vi "Read Math Voltage.vi"(8 "error in (no error)":errorcluster, 11 "VISA resource name":refnum<visa-resource-name>) -> (0 "error out":errorcluster, 2 "amplitude":dbl format="%.2p", 3 "VISA resource name out":refnum<visa-resource-name>)   [LabVIEW 2017]
doc: "You need to run the Initilize.Vi and the Close.vi for the Oscilloscope before and after this Vi. This doens't include those for the sake of runtime."
uses:
  <instrlib>/Tektronix TDS 200 1000 2000 Series/Public/Data/Read (Single Waveform).vi
  <vilib>/measure/mascope.llb/Amplitude and Levels 1 chan.vi
  <instrlib>/Tektronix TDS 200 1000 2000 Series/Tektronix TDS 200 1000 2000 Series.lvlib
  <vilib>/measure/NI_MAPro.lvlib
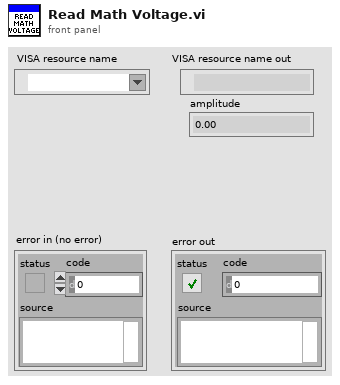
[diagram p1: front panel]
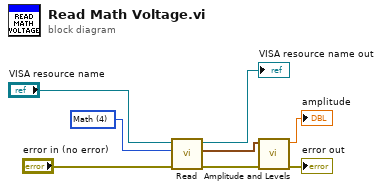
[diagram p0: block diagram]
diagram:
  w7 = u16 4 items=["Channel 1", "Channel 2", "Channel 3", "Channel 4", "Math", "Reference A", "Reference B", "Reference C", "Reference D", "FFT"] ("Source (0: Channel 1)")
  n1 = call-poly <instrlib>:"Read.vi"("error in (no error)"="error in (no error)", "Source (0: Channel 1)"=w7, "VISA resource name"="VISA resource name") -> ("error out"=w3:errorcluster, "Waveform Data"=w4:waveform(dbl), "VISA resource name out"=→"VISA resource name out":refnum<visa-resource-name>)  [unwired: 6 in]
  n2 = call-poly <vilib>:"Amplitude and Levels.vi"("error in (no error)"=w3, "signal in"=w4) -> ("error out"=→"error out":errorcluster, "amplitude"=→"amplitude":dbl)  [unwired: 6 in, 2 out]
